vi "Actor Core.vi"(8 "error in":errorcluster, 11 "ViewableOne In":refnum<class "ViewableOne.lvclass">) -> (0 "error out":errorcluster, 3 "Actor out":refnum<class "Actor.lvclass">)   [LabVIEW 2017, in "ViewableDoubles.lvlib" / "ViewableOne.lvclass"]
doc: "(<B>Filename</B>: Actor Framework.lvlib:Actor.lvclass:Actor Core.vi)\n\nReceives messages to the actor, reacts to them, and initiates any error handling that may shut the actor down.\n\nDescendant classes may override this VI to append parallel tasks for the actor to complete while it handles messages. Overrides use the Call Parent Method node.\n\n<License>\nCopyright © 2017 Composed Systems, LLC | All rights reserved\nwww.composed.io\n\nAuthor: Ethan Stern <ethan.stern@composed.io>\n\nThis software is provided \"AS IS\" WITHOUT WARRANTIES, either express or implied, AND IS FOR EDUCATIONAL PURPOSES ONLY.\n</License>"
uses:
  ViewableOne.lvclass
  <vilib>/ActorFramework/Actor/Actor.lvclass
  LeakyViewable/LeakyViewable.lvclass
panel:
  # "ViewableOne"
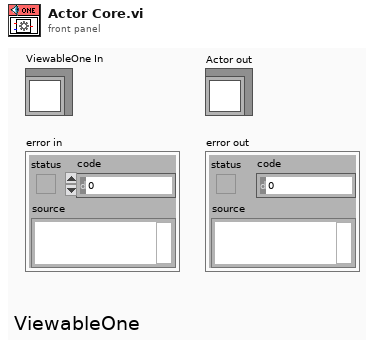
[diagram p1: front panel]
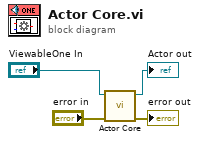
[diagram p0: block diagram]
diagram:
  n1 = call-parent "Actor Core.vi"("error in"="error in", "LeakyViewable In"="ViewableOne In") -> ("error out"=→"error out":errorcluster, "Actor out"=→"Actor out":refnum<class "Actor.lvclass">)  [unwired: 8 in]
